vi "updateBuffer.vi"(9 "Buffer size":i32, 10 "New elements":bool[](array[boolean])=[FALSE], 11 "Buffer in":bool[](array[boolean])=[FALSE]) -> (3 "Updated buffer":bool[](array[boolean]))   [LabVIEW 2017]
doc: "Update buffer (array) with new elements, trimming to buffer size if necessary"
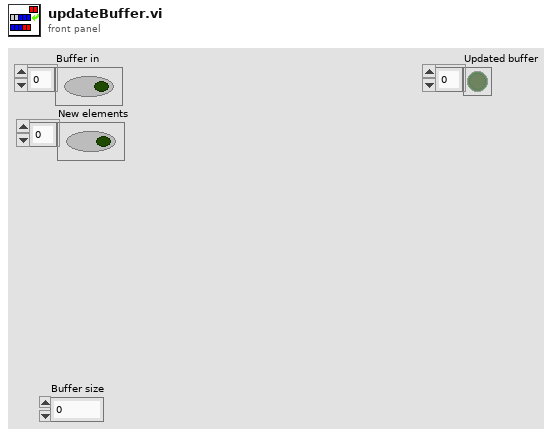
[diagram p1: front panel]
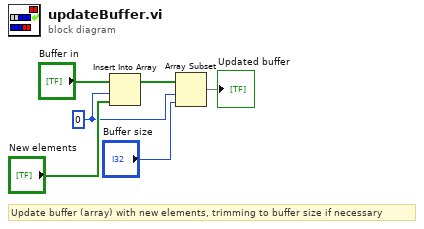
[diagram p0: block diagram]
diagram:
  w3 = 0 ("index")
  # "Update buffer (array) with new elements, trimming to buffer size if necessary"
  n1 = Insert Into Array(array="Buffer in", index=w3, new element="New elements") -> (w4:bool[])
  n2 = Array Subset(array=w4, index=w3, length="Buffer size") -> (→"Updated buffer":bool[])
